vi "Configure Frequency.vi"(7 "Mode":enum16{"Center Span", "Start Stop"}(ring), 8 "error in (no error)":errorcluster, 9 "Span/Stop Frequency":dbl, 10 "Center/Start Frequency":dbl, 11 "VNA-ENA in":refnum<class "VNA-ENA.lvclass">) -> (0 "error out":errorcluster, 3 "VNA-ENA out":refnum<class "VNA-ENA.lvclass">)   [LabVIEW 2020, in "VNA-ENA.lvclass"]
doc: "Configures the frequency range for the sweep.\nThe default mode is Center Span."
uses:
  VNA-ENA.lvclass
  C:/Sandbox/Git_Sandbox/WiSpry Test Framework source code (LV20)/WiSpry Test Framework/Instruments/Instrument.lvclass
  Instrument.lvclass/Instrument.ctl
  Instrument.lvclass
  <instrlib>/Agilent ENA Series/Agilent ENA Series.lvlib
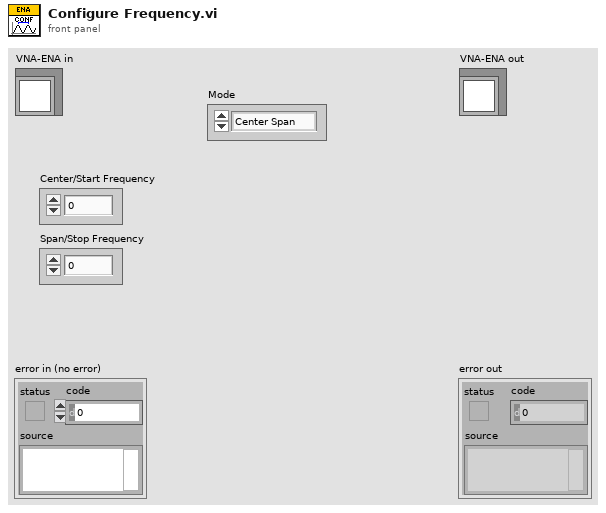
[diagram p1: front panel]
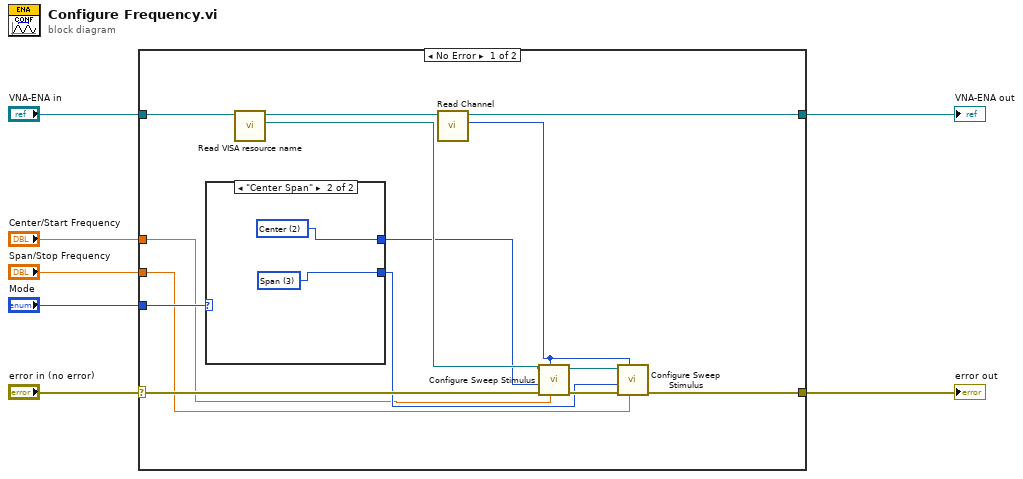
[diagram p0: block diagram]
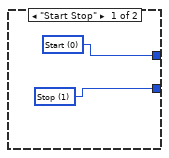
[diagram p2: hidden frame]
diagram:
  n1 = case shown="No Error" "error in (no error)" {
    selector: "error in (no error)" -> [w17 w27]
    tunnel: [w15 w27] -> w7
    tunnel: [w18 w26] -> w6
    tunnel: "VNA-ENA in" -> [w21 w26]
    tunnel: "Mode" -> [w20 _]
    tunnel: "Center/Start Frequency" -> [w8 _]
    tunnel: "Span/Stop Frequency" -> [w9 _]
    frame No Error {
      n2 = case shown="\"Center Span\"" w20 {
        tunnel: [w23 w25] -> w10
        tunnel: [w22 w24] -> w11
        frame "Start Stop" {
          w22 = u16 1 items=["Start", "Stop", "Center", "Span"] ("Stimulus (0: Start)")
          w23 = u16 0 items=["Start", "Stop", "Center", "Span"] ("Stimulus (0: Start)")
        }
        frame "Center Span" {
          w24 = u16 3 items=["Start", "Stop", "Center", "Span"] ("Stimulus (0: Start)")
          w25 = u16 2 items=["Start", "Stop", "Center", "Span"] ("Stimulus (0: Start)")
        }
      }
      n3 = call "Read VISA resource name.vi"("Instrument in"=w21) -> ("VISA resource name"=w13:refnum<visa-resource-name>, "Instrument out"=w19:refnum<class "VNA-ENA.lvclass">)  [unwired: 9 in]
      n4 = call-dynamic "Read Channel.vi"("Vector Network Analyzer in"=w19) -> ("Channel"=w12:i32, "Vector Network Analyzer out"=w18:refnum<class "VNA-ENA.lvclass">)  [unwired: 9 in]
      n5 = call <instrlib>:"Configure Sweep Stimulus.vi"("Parameter (0.0)"=w8, "Channel (1)"=w12, "error in (no error)"=w17, "Stimulus (0: Start)"=w10, "VISA resource name"=w13) -> ("error out"=w16:errorcluster, "VISA resource name out"=w14:refnum<visa-resource-name>)  [unwired: 5 in]
      n6 = call <instrlib>:"Configure Sweep Stimulus.vi"("Parameter (0.0)"=w9, "Channel (1)"=w12, "error in (no error)"=w16, "Stimulus (0: Start)"=w11, "VISA resource name"=w14) -> ("error out"=w15:errorcluster)  [unwired: 5 in, 1 out]
    }
    frame Error {
    }
  }
  "error out" <- w7
  "VNA-ENA out" <- w6
